vi "From Json.vi"(7 "Package Folder":path, 8 "error in (no error)":errorcluster, 11 "JSON in":string) -> (0 "error out":errorcluster, 3 "Package out":refnum<class "Package.lvclass">)   [LabVIEW 2020, in "neg-pkg.lvlib" / "Package.lvclass"]
uses:
  Package.lvclass
  semver/Semver/Semver.lvclass/Semver.ctl
  Package.lvclass/Package.ctl
  semver/Semver/Parse Number.vi
  <vilib>/Utility/error.llb/Error Cluster From Error Code.vi
  semver/Semver/Semver.lvclass
  neg_pkgs/negentropicdev/lv-json/JSON/JSON.lvlib
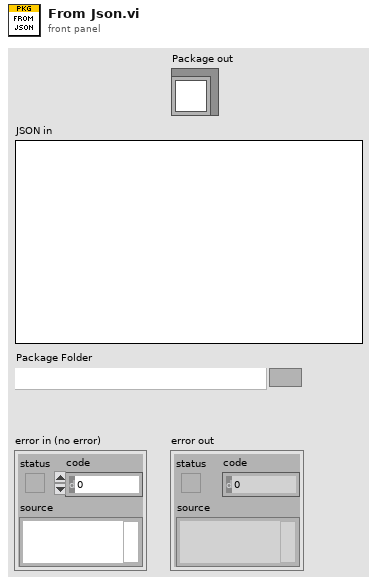
[diagram p1: front panel]
types:
  T1 = typedef "JSON.lvlib/JSON Item Type.ctl" = enum16{"unknown", "null", "Array", "Object", "String", "Number", "Boolean"}
  T2 = typedef "neg-pkg.lvlib/Package.lvclass/Package ID.ctl" = cluster{"Type":T3, "Scope":string, "Name":string, "Resource":string}
  T3 = typedef "neg-pkg.lvlib/Package.lvclass/Package Type.ctl" = enum16{"unspecified", "git"}
  T4 = typedef "neg-pkg.lvlib/Package.lvclass/Dependency.ctl" = cluster{"Package":T2, "Version":string}
  T5 = typedef "neg-pkg.lvlib/Package.lvclass/Build Item.ctl" = cluster{"Project":path, "Target":string, "Build Spec":string}
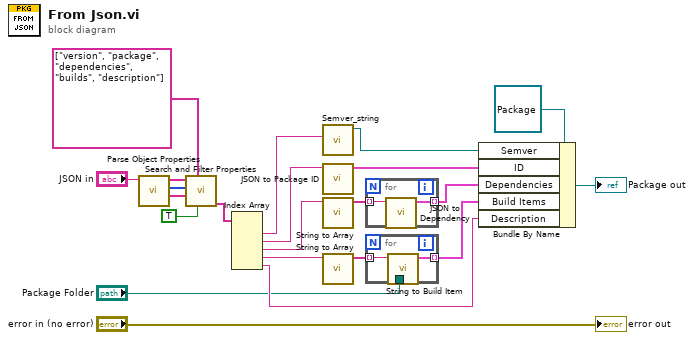
[diagram p0: block diagram]
diagram:
  n1 = call "Parse Object Properties.vi"("JSON String"="JSON in") -> ("Values"=w18:string[], "Item Types"=w19:T1[], "Keys"=w20:string[])  [unwired: 7 in, 1 out]
  n2 = call "Search and Filter Properties.vi"("Remove Found? (F)"=TRUE, "Search Keys"=string[] ["version", "package", "dependencies", "builds", "description"], "Values In"=w18, "Types In"=w19, "Keys In"=w20) -> ("Filtered Values"=w15:string[])  [unwired: 1 in, 5 out]
  n3 = Index Array(array=w15) -> (element #1=w9:string, element #2=w8:string, element #3=w14:string, element #4=w13:string, element #5=w4:string)  [unwired: 5 in]
  n4 = call "Semver_string.vi"("Version"=w9) -> ("Semver out"=w6:refnum<class "Semver.lvclass">)  [unwired: 9 in, 1 out]
  n5 = call "JSON to Package ID.vi"("JSON"=w8) -> ("Package"=w7:T2)  [unwired: 10 in]
  n6 = call "String to Array.vi"("Array String In"=w14) -> ("JSON Strings"=w12:string[])  [unwired: 10 in]
  n7 = call "String to Array.vi"("Array String In"=w13) -> ("JSON Strings"=w3:string[])  [unwired: 10 in]
  n8 = for {
    tunnel: w12 -> [w24] mode=indexing
    tunnel: [w23] -> w5 mode=indexing
    n9 = call "JSON to Dependency.vi"("Dependency JSON"=w24) -> ("Dependency"=w23:T4)  [unwired: 10 in]
  }
  n10 = for {
    tunnel: w3 -> [w27] mode=indexing
    tunnel: "Package Folder" -> [w26]
    tunnel: [w25] -> w1 mode=indexing
    n11 = call "String to Build Item.vi"("Package Folder"=w26, "String"=w27) -> ("Build Item"=w25:T5)  [unwired: 9 in]
  }
  n12 = Bundle By Name(cluster=refnum<class "Package.lvclass"> refnum ("Package out"), "Semver"=w6, "ID"=w7, "Dependencies"=w5, "Build Items"=w1, "Description"=w4) -> (→"Package out":refnum<class "Package.lvclass">)
  "error out" <- "error in (no error)"
